vi "Get Item Property (Dependent Node Pointer).vi"(8 "error in (no error)":errorcluster, 10 "Property Name":string, 11 "Item Ref in":T1 format="%.0x") -> (0 "error out":errorcluster, 1 "Dependent Node Ref":T1=18446744073709551615 format="%.0x", 3 "Item Ref out":T1 format="%.0x", 4 "Found":bool)   [LabVIEW 2026, in "Custom Devices Storage.lvlib"]
uses:
  Custom Devices Storage.lvlib
  <vilib>/NI VeriStand/Custom Device API/Custom Device Item Ref.ctl
  C:/Users/Administrator/Desktop/Jatin/All DNC DLLs/NationalInstruments.VeriStand.SystemDefinitionAPI.dll
  Jatin/All DNC DLLs/NationalInstruments.VeriStand.SystemDefinitionAPI.dll
  <vilib>/NI VeriStand/Custom Device API/Custom Device API.lvlib
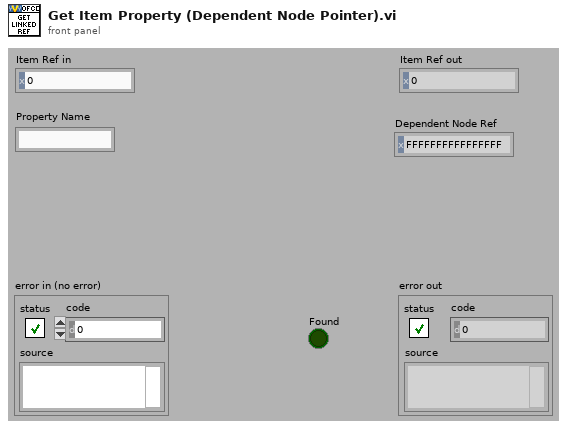
[diagram p1: front panel]
types:
  T1 = typedef "Custom Device API.lvlib/Custom Device Item Ref.ctl" = u64
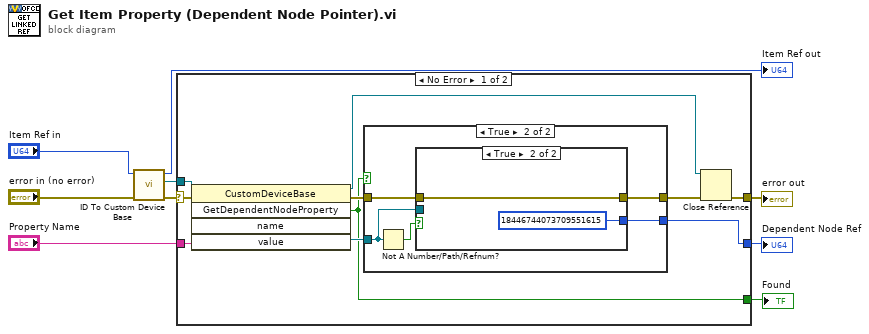
[diagram p0: block diagram]
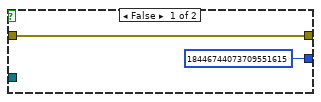
[diagram p2: hidden frame]
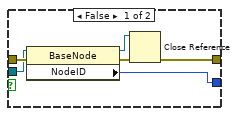
[diagram p3: hidden frame]
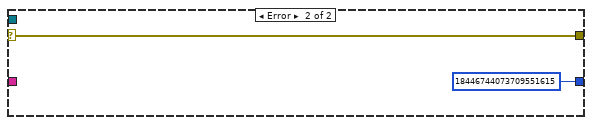
[diagram p4: hidden frame]
diagram:
  n1 = call "ID To Custom Device Base.vi"("error in (no error)"="error in (no error)", "ID in"="Item Ref in") -> ("error out"=w7:errorcluster, "NationalInstruments.VeriStand.SystemDefinitionAPI.CustomDeviceBase"=w6:refnum<k39>, "ID out"=→"Item Ref out":u64)  [unwired: 7 in]
  n2 = case shown="No Error" w7 {
    selector: w7 -> [w18 w36]
    tunnel: w6 -> [w19 _]
    tunnel: "Property Name" -> [w17 _]
    tunnel: [w14 T1 18446744073709551615 ("Dependent Node Ref")] -> w4
    tunnel: [w11 w36] -> w3
    tunnel: [w10 _] -> w2
    frame No Error {
      n3 = invoke class="CustomDeviceBase" method="GetDependentNodeProperty"(reference=w19, error in=w18, "name"=w17) -> (reference out=w12:refnum<k39>, error out=w15:errorcluster, "GetDependentNodeProperty"=w10:bool, "value"=w16:refnum<k39>)  [unwired: 2 in, 1 out]
      n4 = case shown="True" w10 {
        tunnel: w16 -> [_ w25]
        tunnel: w15 -> [w21 w26]
        tunnel: [T1 18446744073709551615 ("Dependent Node Ref") w23] -> w14
        tunnel: [w21 w22] -> w13
        frame False {
        }
        frame True {
          n5 = Not A Number/Path/Refnum?(number/path/refnum=w25) -> (NaN/Path/Refnum?=w24:bool)
          n6 = case shown="True" w24 {
            tunnel: w26 -> [w32 w33]
            tunnel: w25 -> [w31 _]
            tunnel: [w30 T1 18446744073709551615 ("Dependent Node Ref")] -> w23
            tunnel: [w27 w33] -> w22
            frame False {
              n7 = property class="BaseNode"(reference=w31, error in=w32) -> (reference out=w28:refnum<k39>, error out=w29:errorcluster, "NodeID"=w30:u64)
              n8 = Close Reference(reference=w28, error in (no error)=w29) -> (error out=w27:errorcluster)
            }
            frame True {
            }
          }
        }
      }
      n9 = Close Reference(reference=w12, error in (no error)=w13) -> (error out=w11:errorcluster)
    }
    frame Error {
    }
  }
  "error out" <- w3
  "Found" <- w2
  "Dependent Node Ref" <- w4
